vi "XW_Create_Map_tf.vi"() -> ()   [LabVIEW 2021]
uses:
  Controls/Cal_Inst_type.ctl
  <vilib>/Utility/file.llb/Write To Spreadsheet File (DBL).vi
  Controls/File_Selector_Type.ctl
  <vilib>/Analysis/NI_AALBase.lvlib
  <vilib>/Analysis/baseanly.llb/Mean (DBL).vi
panel:
  out "Velocity Points":dbl[][](array[numeric])
  out "index of element":i32
  out "2D data array":dbl[][](array[numeric]) format="%.2f"
  out "Off 2":dbl
  out "Gain 2":dbl
  out "Off 1":dbl
  out "Gain 1":dbl
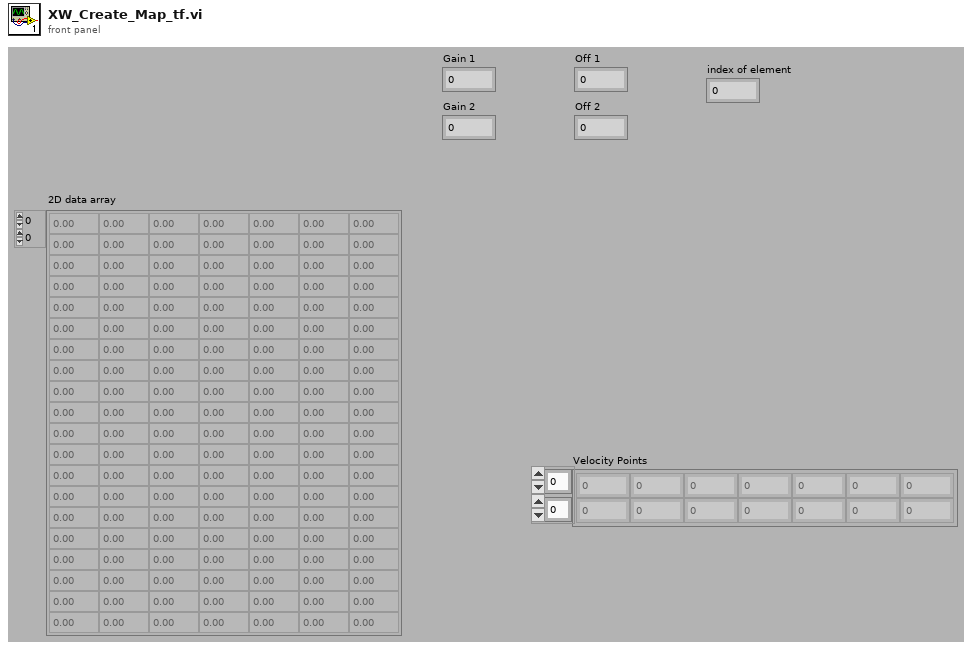
[diagram p1: front panel]
types:
  T1 = typedef "File_Selector_Type.ctl" = enum16{"The Selected File", "The Selected Folder", "Files containing the search string in the selected folder", "All files listed in selected file"}
  T2 = typedef "Cal_Inst_type.ctl" = enum16{"Propeller anemometer", "Pressure Transducer", "Hot wire", "Cross wire velocity", "Cross wire angle", "Generic Linear", "Generic Polynomial", "Poly Fit Special", "Fast FID", "Thermocouple", "Cold wire", "Pulsed Wire"}
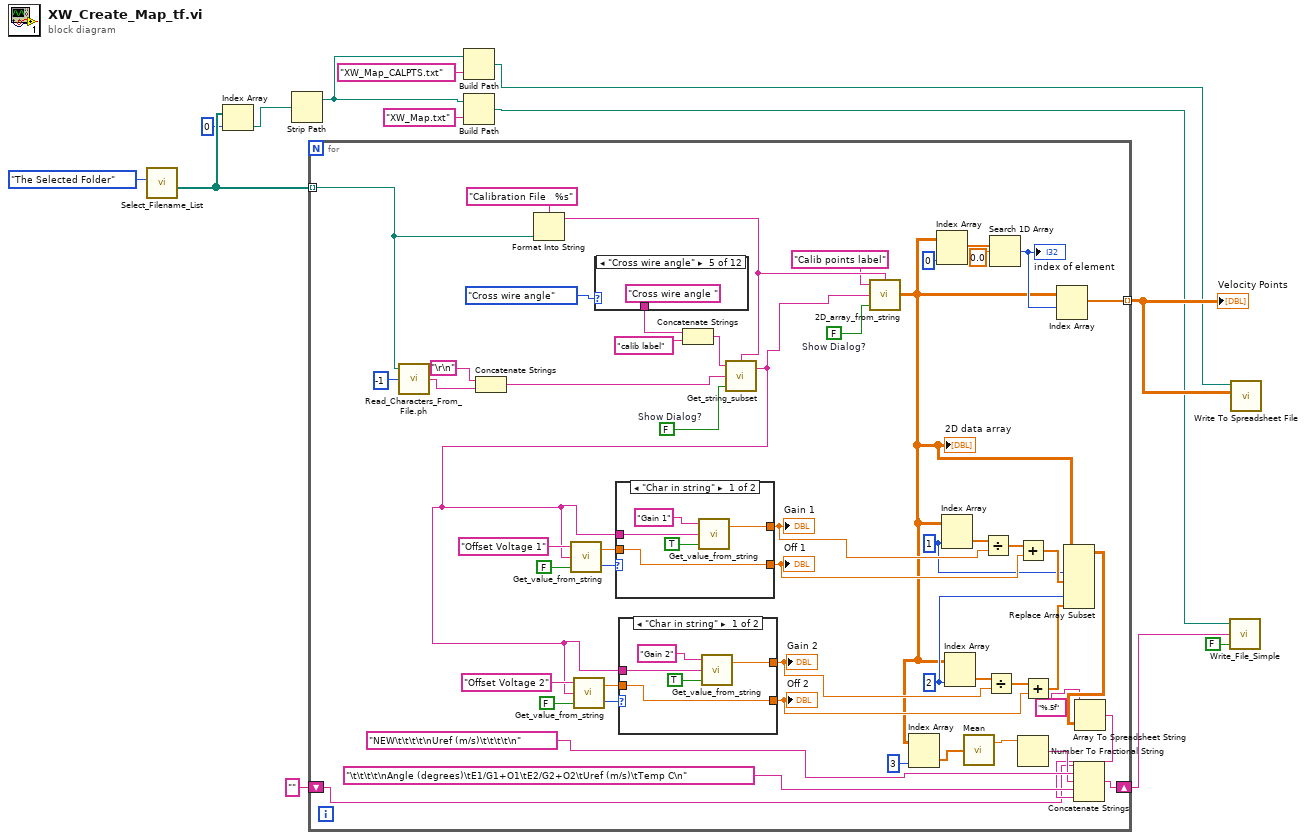
[diagram p0: block diagram]
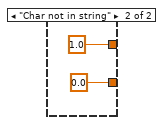
[diagram p2: hidden frame]
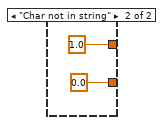
[diagram p3: hidden frame]
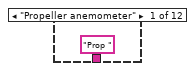
[diagram p4: hidden frame]
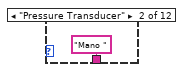
[diagram p5: hidden frame]
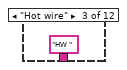
[diagram p6: hidden frame]
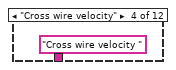
[diagram p7: hidden frame]
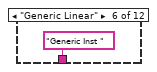
[diagram p8: hidden frame]
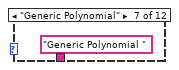
[diagram p9: hidden frame]
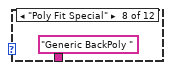
[diagram p10: hidden frame]
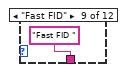
[diagram p11: hidden frame]
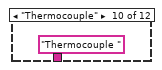
[diagram p12: hidden frame]
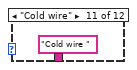
[diagram p13: hidden frame]
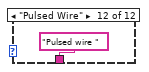
[diagram p14: hidden frame]
diagram:
  n1 = call "Select_Filename_List.vi"("At Dialog Prompt Post Process"=File_Selector_Type."The Selected Folder") -> ("Selected files"=w8:path[])  [unwired: 5 in, 2 out]
  n2 = Index Array(array=w8, index=0) -> (element=w6:path)
  n3 = Strip Path(path=w6) -> (stripped path=w3:path)  [unwired: 1 out]
  n4 = for {
    tunnel: w8 -> [w44] mode=indexing
    tunnel: [w38] -> w13 mode=indexing
    shift-right: [w14] -> w11
    shift-left: "" -> [w15]
    w27 = 2 ("index (col)")
    w28 = 1 ("index (col)")
    w55 = FALSE  # Show Dialog?
    w63 = FALSE  # Show Dialog?
    n5 = call "Read_Characters_From_File.ph.vi"("file path (dialog if empty)"=w44, "number of characters (all:-1)"=-1) -> ("character string"=w65:string)  [unwired: 7 out]
    n6 = Concatenate Strings("\r\n", w65) -> (w45:string)
    n7 = Format Into String(format string="Calibration File   %s", w44) -> (resulting string=w57:string)  [unwired: 2 in, 1 out]
    n8 = case shown="\"Cross wire angle\"" Cal_Inst_type."Cross wire angle" ("Instrument type") {
      tunnel: ["Prop " "Mano " "HW " "Cross wire velocity " "Cross wire angle " "Generic Inst " "Generic Polynomial " "Generic BackPoly " "Fast FID " "Thermocouple " "Cold wire " "Pulsed wire "] -> w62
      frame "Propeller anemometer" {
      }
      frame "Pressure Transducer" {
      }
      frame "Hot wire" {
      }
      frame "Cross wire velocity" {
      }
      frame "Cross wire angle" {
      }
      frame "Generic Linear" {
      }
      frame "Generic Polynomial" {
      }
      frame "Poly Fit Special" {
      }
      frame "Fast FID" {
      }
      frame "Thermocouple" {
      }
      frame "Cold wire" {
      }
      frame "Pulsed Wire" {
      }
    }
    n9 = Concatenate Strings(w62, "calib label") -> (w61:string)
    n10 = call "Get_string_subset.vi"("String Name"=w57, "Show Dialog?"=w63, "String to split"=w45, "File Label"=w61) -> ("Output string"=w43:string)  [unwired: 1 out]
    n11 = call "Get_value_from_string.vi"("Show Dialog?"=FALSE, "Input string"=w43, "Variable name"="Offset Voltage 1") -> ("Status"=w51:enum16{"Char in string", "Char not in string"}, "Value"=w50:dbl)
    n12 = call "Get_value_from_string.vi"("Show Dialog?"=FALSE, "Input string"=w43, "Variable name"="Offset Voltage 2") -> ("Status"=w48:enum16{"Char in string", "Char not in string"}, "Value"=w49:dbl)
    n13 = case shown="\"Char in string\"" w51 {
      tunnel: w43 -> [w77 _]
      tunnel: [w74 1.0 ("Value")] -> w31
      tunnel: w50 -> [w73 _]
      tunnel: [w73 0.0 ("Value")] -> w30
      frame "Char in string" {
        n14 = call "Get_value_from_string.vi"("Show Dialog?"=TRUE, "Input string"=w77, "Variable name"="Gain 1") -> ("Value"=w74:dbl)  [unwired: 1 out]
      }
      frame "Char not in string" {
      }
    }
    "Gain 1" <- w31
    "Off 1" <- w30
    n15 = case shown="\"Char in string\"" w48 {
      tunnel: w43 -> [w70 _]
      tunnel: [w67 1.0 ("Value")] -> w36
      tunnel: w49 -> [w66 _]
      tunnel: [w66 0.0 ("Value")] -> w35
      frame "Char in string" {
        n16 = call "Get_value_from_string.vi"("Show Dialog?"=TRUE, "Input string"=w70, "Variable name"="Gain 2") -> ("Value"=w67:dbl)  [unwired: 1 out]
      }
      frame "Char not in string" {
      }
    }
    "Gain 2" <- w36
    "Off 2" <- w35
    n17 = call "2D_array_from_string.vi"("String Name"=w57, "Show Dialog?"=w55, "Input string"=w43, "Array title"="Calib points label") -> ("2D data array"=w25:dbl[][])
    "2D data array" <- w25
    n18 = Index Array(array=w25, index (col)=3 ("disabled index (col)")) -> (element=w23:dbl[])  [unwired: 1 in]
    n19 = Index Array(array=w25, index (col)=0 ("disabled index (col)")) -> (element=w40:dbl[])  [unwired: 1 in]
    n20 = Index Array(array=w25, index (col)=w28) -> (element=w32:dbl[])  [unwired: 1 in]
    n21 = Index Array(array=w25, index (col)=w27) -> (element=w37:dbl[])  [unwired: 1 in]
    n22 = call-poly <vilib>:"Mean.vi"("X"=w23) -> ("mean"=w22:dbl)  [unwired: 1 out]
    n23 = Divide(x=w32, y=w31) -> (x/y=w33:dbl[])
    n24 = Divide(x=w37, y=w36) -> (x/y=w34:dbl[])
    n25 = Search 1D Array(1D array=w40, element=0.0) -> (index of element=w39:i32)  [unwired: 1 in]
    "index of element" <- w39
    n26 = Add(x=w33, y=w30) -> (x+y=w29:dbl[])
    n27 = Number To Fractional String(number=w22) -> (F-format string=w20:string)  [unwired: 3 in]
    n28 = Add(x=w34, y=w35) -> (x+y=w26:dbl[])
    n29 = Index Array(array=w25, index (row)=w39) -> (element=w38:dbl[])  [unwired: 1 in]
    n30 = Replace Array Subset(array=w25, new element #1=w29, index (col) #1=w28, new element #2=w26, index (col) #2=w27) -> (w18:dbl[][])  [unwired: 2 in]
    n31 = Array To Spreadsheet String(array=w18, 3:"%.5f" ("format string")) -> (spreadsheet string=w16:string)  [unwired: 1 in]
    n32 = Concatenate Strings(w15, "NEW\t\t\t\t\nUref (m/s)\t\t\t\t\n", w20, "\t\t\t\t\nAngle (degrees)\tE1/G1+O1\tE2/G2+O2\tUref (m/s)\tTemp C\n", w16) -> (w14:string)
  }
  "Velocity Points" <- w13
  n33 = Build Path(base path=w3, name or relative path="XW_Map_CALPTS.txt") -> (appended path=w2:path)
  n34 = Build Path(base path=w3, name or relative path="XW_Map.txt") -> (appended path=w1:path)
  n35 = call "Write_File_Simple.vi"("append to file? (new file:F)"=FALSE, "character string"=w11, "file path"=w1) -> ()  [unwired: 2 out]
  n36 = call-poly <vilib>:"Write To Spreadsheet File.vi"("2D data"=w13, "file path (dialog if empty)"=w2) -> ()  [unwired: 6 in, 1 out]
